vi "Polynomial Plot (Range).vi"(8 "P(x)":dbl[](array[numeric]), 9 "end":dbl=1.0, 10 "start":dbl, 11 "samples":i32=100) -> (0 "error":i32, 3 "polynomial plot":cluster{"Ramp Pattern":dbl[], "P(A)":dbl[]}(graph))   [LabVIEW 2020, in "NI_AALPro.lvlib"]
doc: "Plots the evaluations of polynomial <B>P(x)</B>. Wire data to the <B>X</B> input to determine the polymorphic instance to use or manually select the instance."
uses:
  <vilib>/Analysis/NI_AALPro.lvlib
  <vilib>/Analysis/1siggen.llb/Ramp Pattern by Samples.vi
  <vilib>/Analysis/polynomials.llb/1D Polynomial Evaluation (DBL).vi
  <vilib>/Analysis/NI_AALBase.lvlib
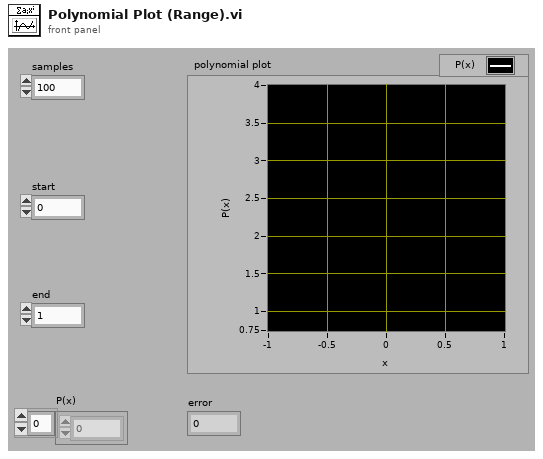
[diagram p1: front panel]
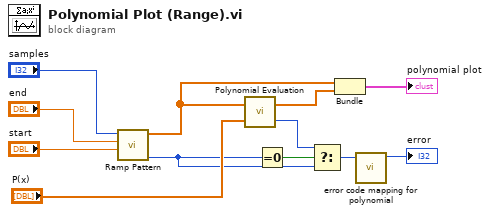
[diagram p0: block diagram]
diagram:
  n1 = call-poly <vilib>:"Ramp Pattern.vi"("start"="start", "end"="end", "samples"="samples") -> ("error"=w4:i32, "Ramp Pattern"=w9:dbl[])  [unwired: 7 in]
  n2 = call-poly <vilib>:"Polynomial Evaluation.vi"("P(x)"="P(x)", "A"=w9) -> ("error"=w5:i32, "P(A)"=w7:dbl[])
  n3 = Equal To 0?(x=w4) -> (x = 0?=w6:bool)
  n4 = Select(t=w5, s=w6, f=w4) -> (s? t:f=w2:i32)
  n5 = Bundle("Ramp Pattern"=w9, "P(A)"=w7) -> (→"polynomial plot":cluster{"Ramp Pattern":dbl[], "P(A)":dbl[]})  [unwired: 1 in]
  n6 = call <vilib>:"error code mapping for polynomial.vi"("error in"=w2) -> ("error out"=→"error":i32)  [unwired: 10 in]
